vi "PSVCH_VI Tree.vi"   [LabVIEW 2016]
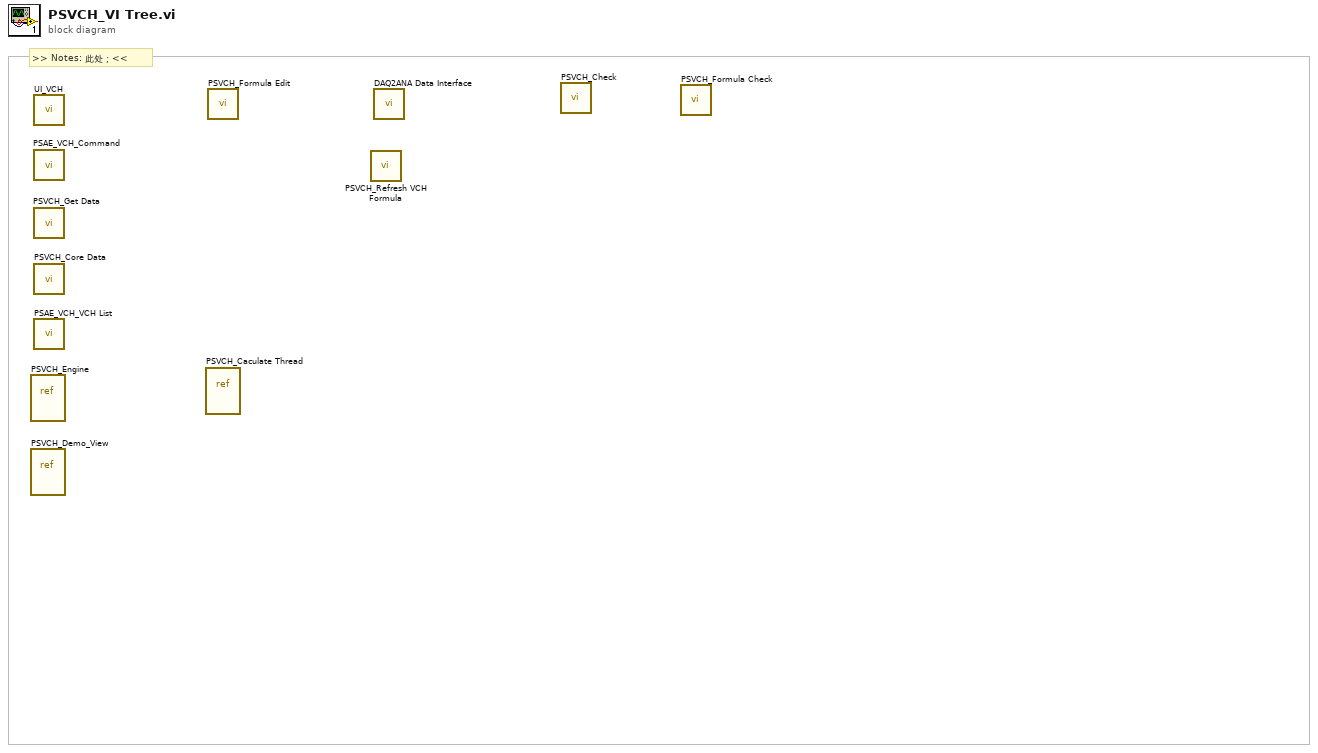
[diagram p0: block diagram]
diagram:
  # ">> Notes: 此处；<<"
  n1 = vi-ref "PSVCH_Engine.vi"() -> ()  [unwired: 1 out]
  n2 = vi-ref "PSVCH_Demo_View.vi"() -> ()  [unwired: 1 out]
  n3 = call "UI_VCH.vi"() -> ()  [unwired: 12 in]
  n4 = call "PSAE_VCH_Command.vi"() -> ()  [unwired: 11 in, 1 out]
  n5 = call "PSVCH_Get Data.vi"() -> ()  [unwired: 9 in, 3 out]
  n6 = call "PSVCH_Core Data.vi"() -> ()  [unwired: 10 in, 2 out]
  n7 = call "PSAE_VCH_VCH List.vi"() -> ()  [unwired: 10 in, 2 out]
  n8 = vi-ref "PSVCH_Caculate Thread.vi"() -> ()  [unwired: 1 out]
  n9 = call "PSVCH_Formula Edit.vi"() -> ()  [unwired: 9 in, 3 out]
  n10 = call "PSVCH_Refresh VCH Formula.vi"() -> ()  [unwired: 10 in, 2 out]
  n11 = call "DAQ2ANA Data Interface.vi"() -> ()  [unwired: 11 in, 1 out]
  n12 = call "PSVCH_Check.vi"() -> ()  [unwired: 9 in, 3 out]
  n13 = call "PSVCH_Formula Check.vi"() -> ()  [unwired: 7 in, 5 out]
